vi "process_project_item.vi"(8 "error in (no error)":errorcluster, 10 "CCSymbols":map{string, string}(c390), 11 "ProjectItem in":refnum<vi>) -> (0 "error out":errorcluster, 3 "ProjectItem out":refnum<vi>)   [LabVIEW 2019]
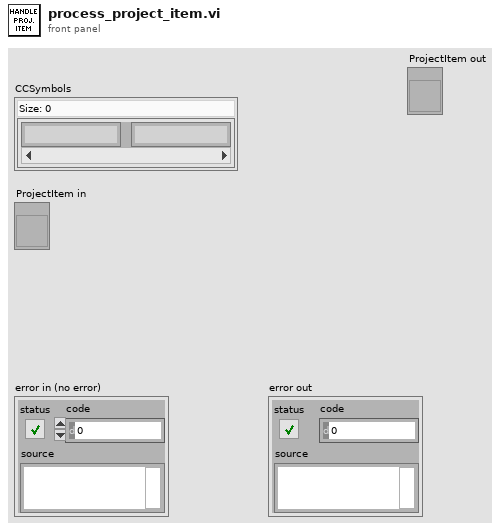
[diagram p1: front panel]
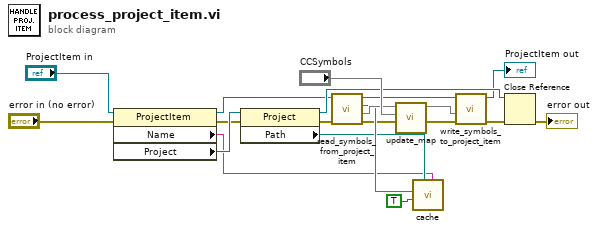
[diagram p0: block diagram]
diagram:
  n1 = property class="ProjectItem"(reference="ProjectItem in", error in="error in (no error)") -> (reference out=w6:refnum<vi>, error out=w5:errorcluster, "Name"=w1:string, "Project"=w9:refnum<vi>)
  n2 = property class="Project"(reference=w9, error in=w5) -> (reference out=w8:refnum<vi>, error out=w4:errorcluster, "Path"=w7:path)
  n3 = call "read_symbols_from_project_item.vi"("error in (no error)"=w4, "ProjectItem in"=w6) -> ("error out"=w11:errorcluster, "CCSymbols"=w14:map{string, string}, "CCSymbols out"=w13:string, "ProjectItem out"=w10:refnum<vi>)  [unwired: 6 in]
  n4 = call "update_map.vi"("New Values"="CCSymbols", "Source"=w14) -> ("Updated"=w15:map{string, string})  [unwired: 9 in]
  n5 = call "cache.vi"("target"=w1, "project path"=w7, "write (T): read (F)"=TRUE, "CCSymbols in"=w13) -> ()  [unwired: 7 in, 1 out]
  n6 = call "write_symbols_to_project_item.vi"("error in (no error)"=w11, "Updated"=w15, "ProjectItem in"=w10) -> ("error out"=w3:errorcluster, "ProjectItem out"=→"ProjectItem out":refnum<vi>)  [unwired: 7 in]
  n7 = Close Reference(reference=w8, error in (no error)=w3) -> (error out=→"error out":errorcluster)
